vi "关键参数交互.vi"() -> ()   [LabVIEW 2016, in "CODCr库.lvlib"]
panel:
  out "x != y?":T1
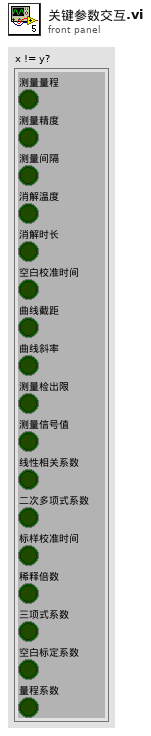
[diagram p1: front panel]
types:
  T1 = cluster{"测量量程":bool, "测量精度":bool, "测量间隔":bool, "消解温度":bool, "消解时长":bool, "空白校准时间":bool, "曲线截距":bool, "曲线斜率":bool, "测量检出限":bool, "测量信号值":bool, "线性相关系数":bool, "二次多项式系数":bool, "标样校准时间":bool, "稀释倍数":bool, "三项式系数":bool, "空白标定系数":bool, "量程系数":bool}
  T2 = cluster{"chose":string, "公式":cluster{"X^2":dbl, "X":dbl, "b":dbl}}
  T3 = cluster{"测量量程":dbl, "测量精度":dbl, "测量间隔":dbl, "消解温度":dbl, "消解时长":dbl, "空白校准时间":timestamp, "曲线截距":dbl, "曲线斜率":dbl, "测量检出限":dbl, "测量信号值":dbl, "线性相关系数":dbl, "二次多项式系数":dbl, "标样校准时间":timestamp, "稀释倍数":dbl, "三项式系数":dbl, "空白标定系数":dbl, "量程系数":dbl}
  T4 = cluster{"时间标识":timestamp, "设备":string, "日志信息":string, "流程参数":string}
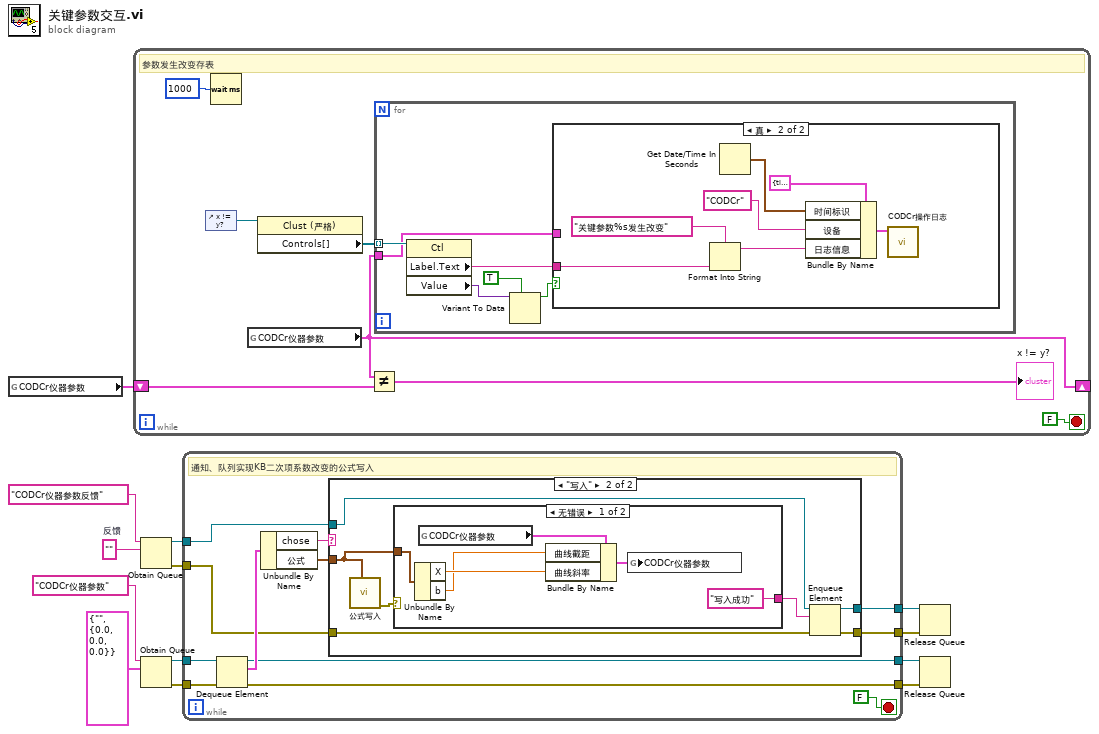
[diagram p0: block diagram]
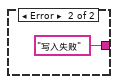
[diagram p3: hidden frame]
diagram:
  w4 = ""  # 反馈
  n1 = global read "CODcr全局变量.vi" "CODCr仪器参数"() -> (w13:T3)
  n2 = while {
    shift-right: [w16] -> _
    shift-left: w13 -> [w18]
    stop <- FALSE stop-if-true
    # "参数发生改变存表"
    n3 = control-ref of="x != y?"() -> (w14:refnum<vi>)
    n4 = Wait (ms)(milliseconds to wait=u32 1000 ("等待时间（毫秒）")) -> ()  [unwired: 1 out]
    n5 = global read "CODcr全局变量.vi" "CODCr仪器参数"() -> (w16:T3)
    n6 = property class="Clust (严格)"(reference=w14) -> ("Controls[]"=w17:refnum<vi>[])  [unwired: 1 in, 2 out]
    n7 = Not Equal?(x=w16, y=w18) -> (x != y?=→"x != y?":T1)
    n8 = for {
      tunnel: w17 -> [w26] mode=indexing
      tunnel: w16 -> [w22]
      n9 = property class="Ctl"(reference=w26) -> ("Label.Text"=w21:string, "Value"=w25:variant)  [unwired: 1 in, 2 out]
      n10 = Variant To Data(type=TRUE, Variant=w25) -> (data=w23:bool)  [unwired: 1 in, 1 out]
      n11 = case shown="真" w23 {
        tunnel: w22 -> [_ _]
        tunnel: w21 -> [_ w31]
        frame False {
        }
        frame True {
          n12 = Format Into String(format string="关键参数%s发生改变" ("格式字符串"), w31) -> (resulting string=w30:string)  [unwired: 2 in, 1 out]
          n13 = Get Date/Time In Seconds() -> (seconds since 1Jan1904=w28:timestamp)
          n14 = Bundle By Name(cluster=T4 {"时间标识"=timestamp(0 s since 1904-01-01), "设备"="", "日志信息"="", "流程参数"=""} ("data in"), "时间标识"=w28, "设备"="CODCr" ("仪器名称"), "日志信息"=w30) -> (w27:T4)
          n15 = call "CODCr操作日志.vi"("data"=w27) -> ()  [unwired: 11 in]
        }
      }
    }
  }
  n16 = Obtain Queue(name (unnamed)="CODCr仪器参数反馈" ("名称（未命名）"), element data type=w4) -> (queue out=w5:refnum<queue>, error out=w3:errorcluster)  [unwired: 3 in, 1 out]
  n17 = Obtain Queue(name (unnamed)="CODCr仪器参数" ("名称（未命名）"), element data type=T2 {"chose"="", "公式"={"X^2"=0.0, "X"=0.0, "b"=0.0}}) -> (queue out=w12:refnum<queue>, error out=w11:errorcluster)  [unwired: 3 in, 1 out]
  n18 = while {
    tunnel: w12 -> [w44]
    tunnel: w11 -> [w43]
    tunnel: [w39] -> w8
    tunnel: [w38] -> w7
    tunnel: w5 -> [w37]
    tunnel: w3 -> [w36]
    tunnel: [w35] -> w2
    tunnel: [w34] -> w1
    stop <- FALSE stop-if-true
    # "通知、队列实现KB二次项系数改变的公式写入"
    n19 = Dequeue Element(queue=w44, error in (no error)=w43) -> (queue out=w39:refnum<queue>, element=w42:T2, error out=w38:errorcluster)  [unwired: 1 in, 1 out]
    n20 = Unbundle By Name(w42) -> ("chose"=w41:string, "公式"=w40:cluster{"X^2":dbl, "X":dbl, "b":dbl})
    n21 = case shown="\"写入\"" w41 {
      tunnel: w40 -> [_ w48]
      tunnel: w37 -> [w47 w54]
      tunnel: w36 -> [w46 w52]
      tunnel: [w47 w51] -> w35
      tunnel: [w46 w50] -> w34
      frame "假", Default {
      }
      frame "写入" {
        n22 = call "公式写入.vi"("公式"=w48) -> ("error out"=w49:errorcluster)  [unwired: 10 in]
        n23 = case shown="无错误" w49 {
          tunnel: ["写入成功" ("消息") "写入失败" ("消息")] -> w53
          tunnel: w48 -> [w57 _]
          frame No Error {
            n24 = Unbundle By Name(w57) -> ("X"=w56:dbl, "b"=w55:dbl)
            n25 = global read "CODcr全局变量.vi" "CODCr仪器参数"() -> (w59:T3)
            n26 = Bundle By Name(cluster=w59, "曲线截距"=w55, "曲线斜率"=w56) -> (w58:T3)
            n27 = global write "CODcr全局变量.vi" "CODCr仪器参数"(w58) -> ()
          }
          frame Error {
          }
        }
        n28 = Enqueue Element(queue=w54, element=w53, error in (no error)=w52) -> (queue out=w51:refnum<queue>, error out=w50:errorcluster)  [unwired: 1 in, 1 out]
      }
    }
  }
  n29 = Release Queue(queue=w2, error in (no error)=w1) -> ()  [unwired: 1 in, 3 out]
  n30 = Release Queue(queue=w8, error in (no error)=w7) -> ()  [unwired: 1 in, 3 out]
